vi "Remove Item.vi"(8 "error in":errorcluster, 11 "Item Ref in":T1 format="%.0x") -> (0 "error out":errorcluster)   [LabVIEW 2026, in "NIVS Runtime Configuration File Scripting API.lvlib"]
uses:
  NIVS Runtime Configuration File Scripting API.lvlib
  <vilib>/NI VeriStand/Custom Device API/Custom Device Item Ref.ctl
  <vilib>/NI VeriStand/Custom Device Offline API/Custom Device Offline API.lvlib
  <vilib>/NI VeriStand/Custom Device API/Custom Device API.lvlib
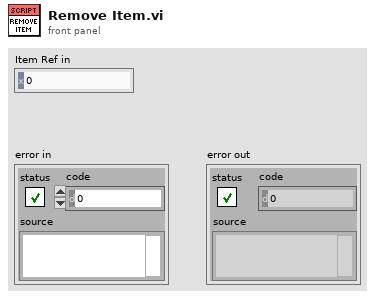
[diagram p1: front panel]
types:
  T1 = typedef "Custom Device API.lvlib/Custom Device Item Ref.ctl" = u64
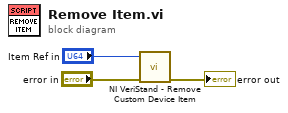
[diagram p0: block diagram]
diagram:
  n1 = call <vilib>:"NI VeriStand - Remove Custom Device Item.vi"("error in (no error)"="error in", "Item Ref in"="Item Ref in") -> ("error out"=→"error out":errorcluster)  [unwired: 8 in, 1 out]
